vi "_get_float.vi"(3 "错误输入（无错误）":errorcluster, 4 "写入缓冲区":string, 5 "VISA资源名称":refnum<visa-resource-name>) -> (0 "错误输出":errorcluster, 1 "数字":sgl, 2 "VISA资源名称输出":refnum<visa-resource-name>)   [LabVIEW 2017]
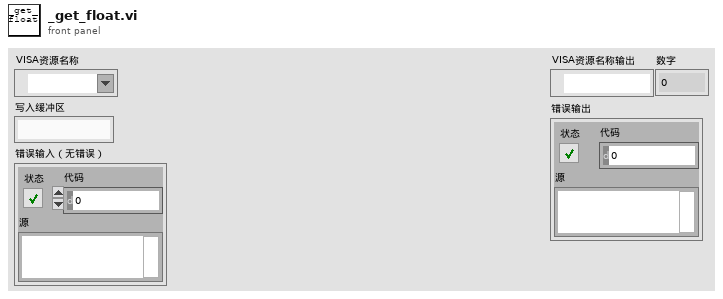
[diagram p1: front panel]
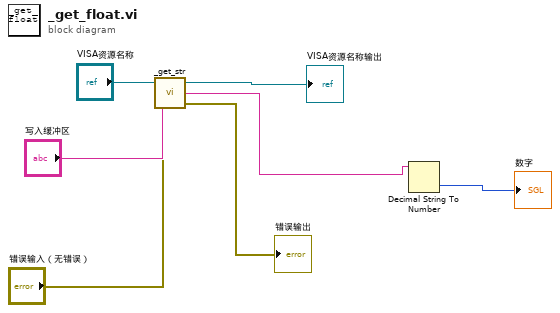
[diagram p0: block diagram]
diagram:
  n1 = call "_get_str.vi"("错误输入（无错误）"="错误输入（无错误）", "写入缓冲区"="写入缓冲区", "VISA资源名称"="VISA资源名称") -> ("错误输出"=→"错误输出":errorcluster, "读取缓冲区"=w2:string, "VISA资源名称输出"=→"VISA资源名称输出":refnum<visa-resource-name>)
  n2 = Decimal String To Number(string=w2) -> (number=→"数字":i32)  [unwired: 2 in, 1 out]
